vi "SetClassRef.vi"(8 "error in (no error)":errorcluster, 10 "FAMM.lvclass":refnum<class "FAMM.lvclass">, 11 "FAMM in":refnum<class "FAMM.lvclass">) -> (0 "error out":errorcluster, 3 "FAMM out":refnum<class "FAMM.lvclass">)   [LabVIEW 2020, in "Sgraph_lib_V1.lvlib" / "FAMM.lvclass"]
doc: "Write FAMM class Attributes reference.\nOnly needed to point to existing FAMM instance."
uses:
  FAMM.lvclass
  FAMM.lvclass/FAMM.ctl
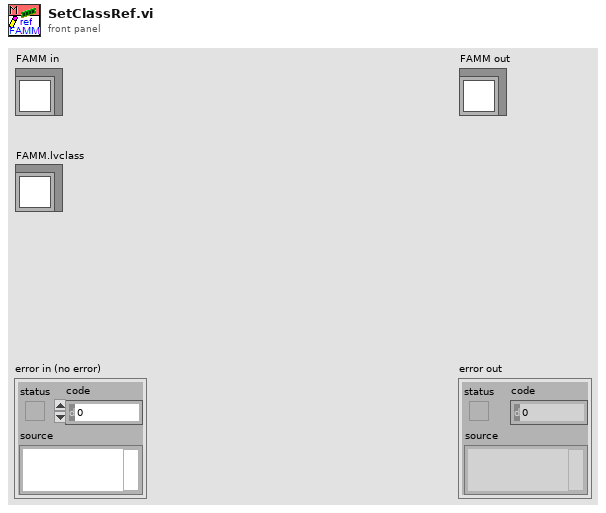
[diagram p1: front panel]
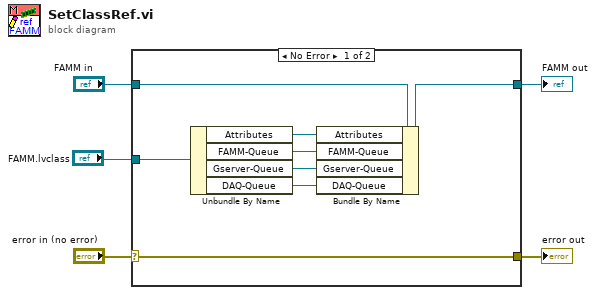
[diagram p0: block diagram]
diagram:
  n1 = case shown="No Error" "error in (no error)" {
    selector: "error in (no error)" -> [w13 w14]
    tunnel: [w13 w14] -> w4
    tunnel: [w12 w15] -> w2
    tunnel: "FAMM in" -> [w11 w15]
    tunnel: "FAMM.lvclass" -> [w10 _]
    frame No Error {
      n2 = Unbundle By Name(w10) -> ("Attributes"=w9:refnum<data-value>, "FAMM-Queue"=w8:refnum<queue>, "Gserver-Queue"=w7:refnum<queue>, "DAQ-Queue"=w6:refnum<queue>)
      n3 = Bundle By Name(cluster=w11, "Attributes"=w9, "FAMM-Queue"=w8, "Gserver-Queue"=w7, "DAQ-Queue"=w6) -> (w12:refnum<class "FAMM.lvclass">)
    }
    frame Error {
    }
  }
  "error out" <- w4
  "FAMM out" <- w2
